vi "PWM Count Controller.vi"(6 "Waveform Generation Mode":fxp<+,2,2> format="%02b", 8 "Enable In":bool, 9 "Counter is Min?":bool, 10 "Counter is Max?":bool, 11 "Reset In":bool) -> (0 "Enable Out":bool, 1 "Direction is Backward?":bool, 2 "Reset Out":bool)   [LabVIEW 2013]
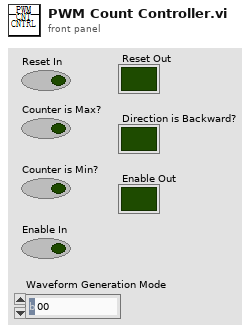
[diagram p1: front panel]
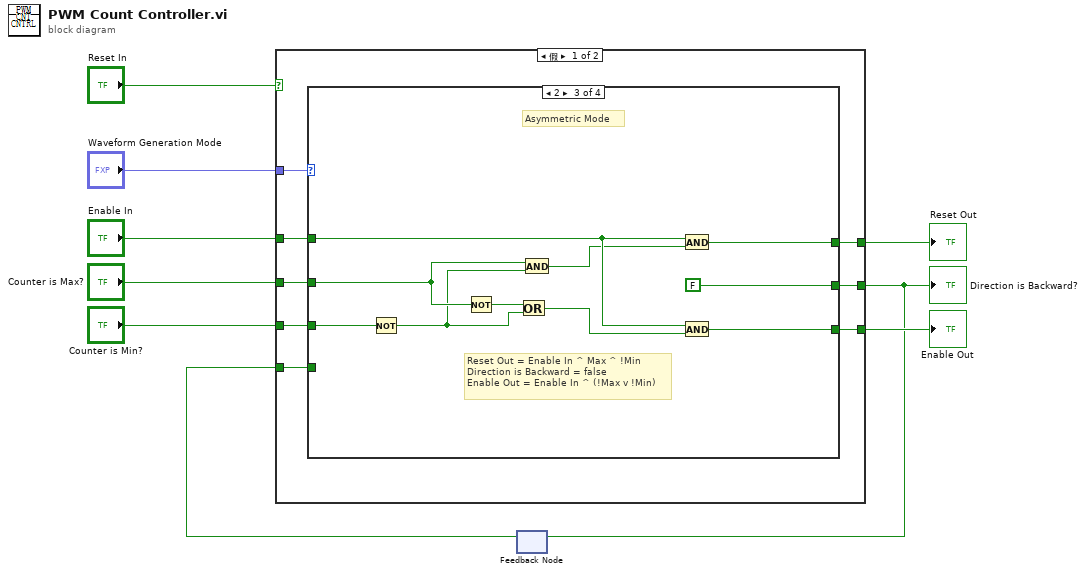
[diagram p0: block diagram]
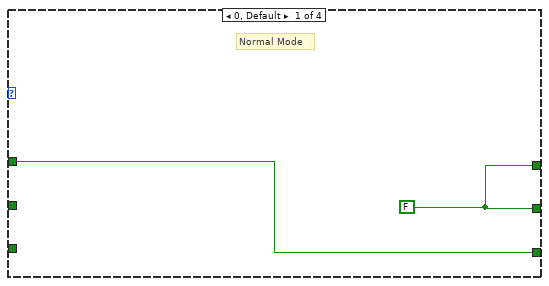
[diagram p2: hidden frame]
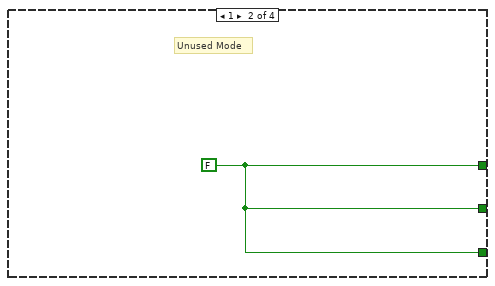
[diagram p3: hidden frame]
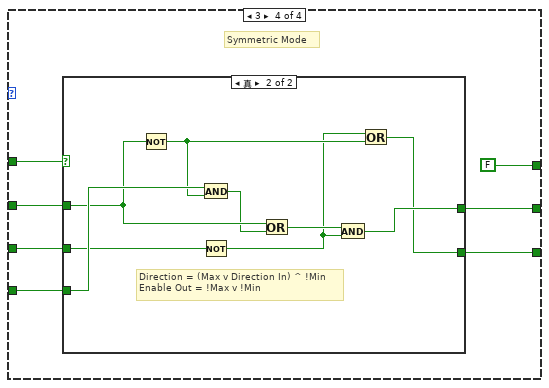
[diagram p4: hidden frame]
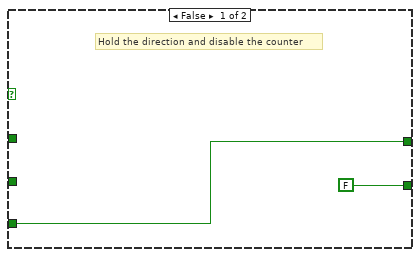
[diagram p5: hidden frame]
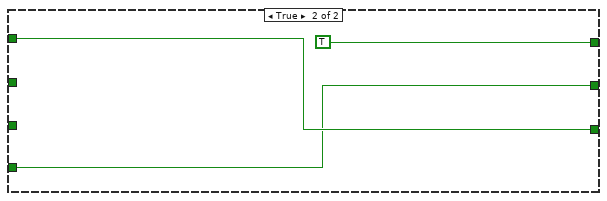
[diagram p6: hidden frame]
diagram:
  n1 = feedback #1() -> (w3:bool)  [unwired: 1 in]
  n2 = case shown="假" "Reset In" {
    tunnel: "Waveform Generation Mode" -> [w17 _]
    tunnel: "Counter is Max?" -> [w16 _]
    tunnel: "Counter is Min?" -> [w15 _]
    tunnel: "Enable In" -> [w14 w50]
    tunnel: [w13 w50] -> w6
    tunnel: [w12 TRUE ("Clock")] -> w5
    tunnel: [w11 w49] -> w4
    tunnel: w3 -> [w10 w49]
    frame False {
      n3 = case shown="2" w17 {
        tunnel: w16 -> [_ _ w28 w35]
        tunnel: w15 -> [_ _ w27 w33]
        tunnel: w14 -> [w18 _ w26 w37]
        tunnel: [w18 w20 w25 w36] -> w13
        tunnel: [w19 w20 w29 FALSE] -> w12
        tunnel: [w19 w20 FALSE w32] -> w11
        tunnel: w10 -> [_ _ _ w34]
        frame 0, Default {
          w19 = FALSE ("Clock")
          # "Normal Mode"
        }
        frame 1 {
          w20 = FALSE ("Clock")
          # "Unused Mode"
        }
        frame 2 {
          # "Reset Out = Enable In ^ Max ^ !Min\nDirection is Backward = false\nEnable Out = Enable In ^ (!Max v !Min)"
          # "Asymmetric Mode"
          n4 = Not(x=w27) -> (.not. x?=w24:bool)
          n5 = Not(x=w28) -> (.not. x?=w23:bool)
          n6 = Or(x=w23, y=w24) -> (x .or. y?=w21:bool)
          n7 = And(x=w28, y=w24) -> (x .and. y?=w22:bool)
          n8 = And(x=w26, y=w22) -> (x .and. y?=w29:bool)
          n9 = And(x=w26, y=w21) -> (x .and. y?=w25:bool)
        }
        frame 3 {
          # "Symmetric Mode"
          n10 = case shown="真" w37 {
            tunnel: w34 -> [w39 w48]
            tunnel: [w39 w43] -> w32
            tunnel: [FALSE w40] -> w36
            tunnel: w35 -> [_ w47]
            tunnel: w33 -> [_ w45]
            frame False {
              # "Hold the direction and disable the counter"
            }
            frame True {
              # "Direction = (Max v Direction In) ^ !Min\nEnable Out = !Max v !Min"
              n11 = Not(x=w47) -> (.not. x?=w42:bool)
              n12 = And(x=w48, y=w42) -> (x .and. y?=w46:bool)
              n13 = Not(x=w45) -> (.not. x?=w41:bool)
              n14 = Or(x=w47, y=w46) -> (x .or. y?=w44:bool)
              n15 = And(x=w44, y=w41) -> (x .and. y?=w43:bool)
              n16 = Or(x=w41, y=w42) -> (x .or. y?=w40:bool)
            }
          }
        }
      }
    }
    frame True {
    }
  }
  "Direction is Backward?" <- w4
  "Reset Out" <- w5
  "Enable Out" <- w6
  n17 = feedback-in #1(w4) -> ()
